vi "BRig_dataCurrent_I_anySelect_L.vi"() -> (2 "output_IanySelect_L":i32)   [LabVIEW 2014]
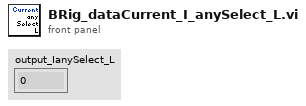
[diagram p1: front panel]
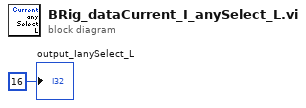
[diagram p0: block diagram]
diagram:
  "output_IanySelect_L" <- 16 ("output_iBlock")
